vi "updatePerturbation.vi"(6 "delta(T)/baseline(F)":bool, 7 "motor":i32, 8 "timeInterval":dbl, 9 "PertSign":i32, 10 "newValue":dbl, 11 "perturbationIn":T1) -> (3 "perturbationOut":T1)   [LabVIEW 2019]
uses:
  TypeDefs/PerturbationControl.ctl
panel:
  # "This VI is used to update the Perturbation Array inserting newValue in the appropriate cell (based on motor axis, pert sign, pert time, delta or baseline)."
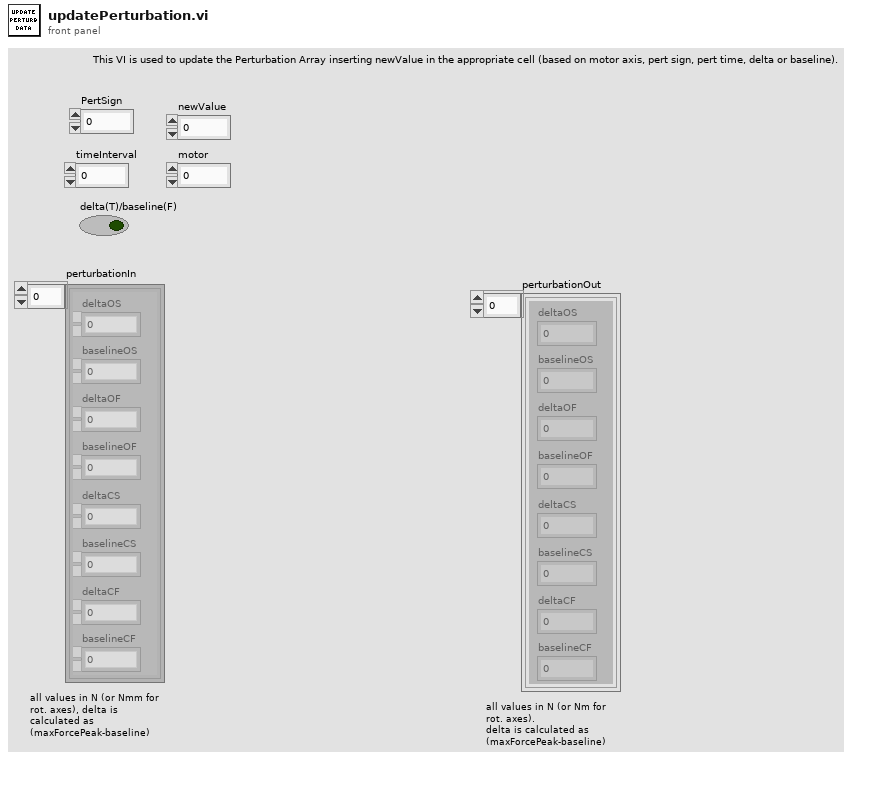
[diagram p1: front panel]
types:
  T1 = typedef "PerturbationControl.ctl" = cluster{"deltaOS":dbl, "baselineOS":dbl, "deltaOF":dbl, "baselineOF":dbl, "deltaCS":dbl, "baselineCS":dbl, "deltaCF":dbl, "baselineCF":dbl}[]
  T2 = cluster{"deltaOS":dbl, "baselineOS":dbl, "deltaOF":dbl, "baselineOF":dbl, "deltaCS":dbl, "baselineCS":dbl, "deltaCF":dbl, "baselineCF":dbl}
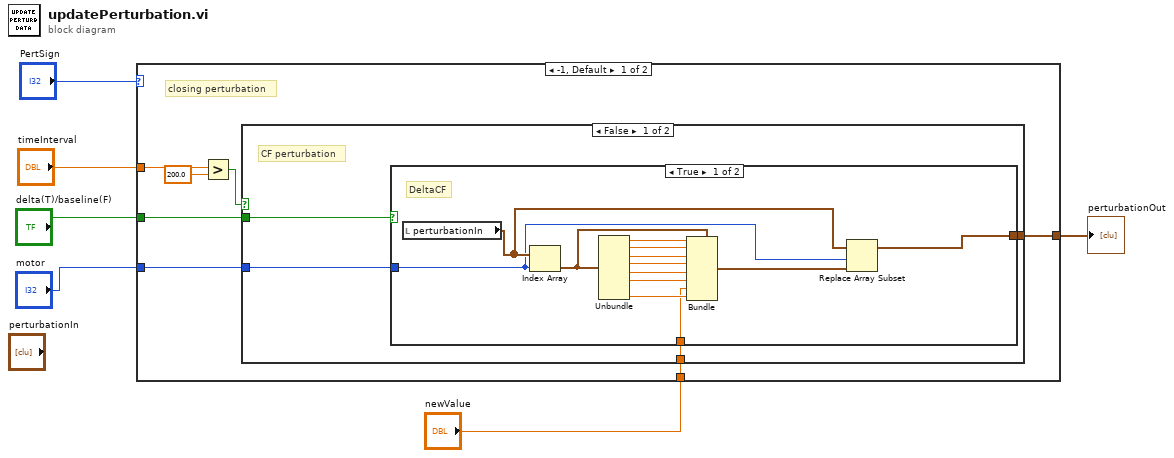
[diagram p0: block diagram]
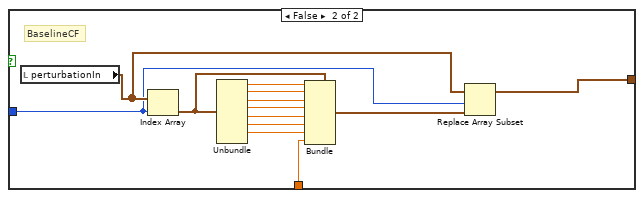
[diagram p2: hidden frame]
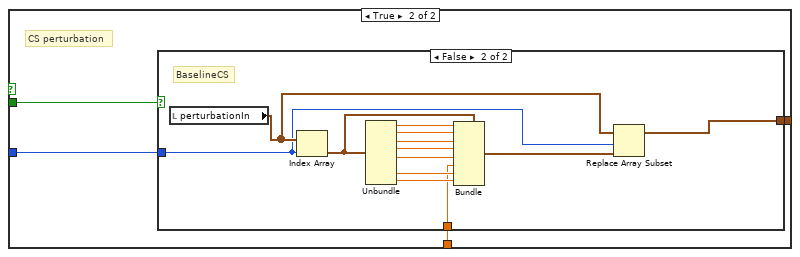
[diagram p3: hidden frame]
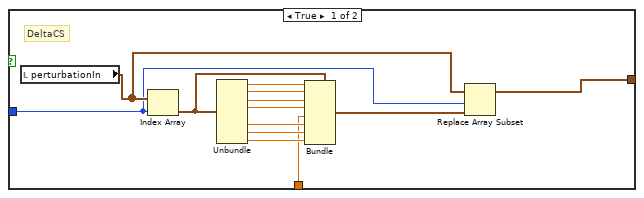
[diagram p4: hidden frame]
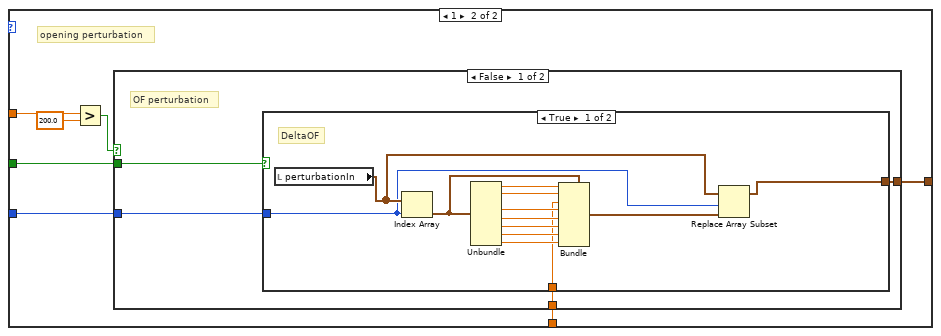
[diagram p5: hidden frame]
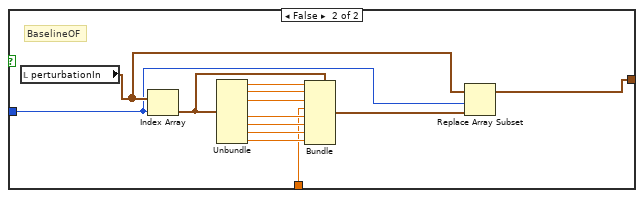
[diagram p6: hidden frame]
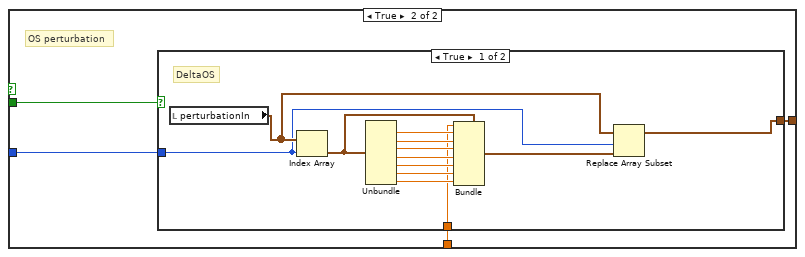
[diagram p7: hidden frame]
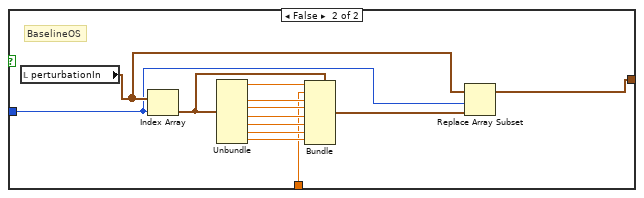
[diagram p8: hidden frame]
diagram:
  n1 = case shown="-1, Default" "PertSign" {
    tunnel: "timeInterval" -> [w13 w80]
    tunnel: "delta(T)/baseline(F)" -> [w10 w77]
    tunnel: "motor" -> [w9 w76]
    tunnel: "newValue" -> [w8 w75]
    tunnel: [w7 w74] -> w1
    frame -1, Default {
      # "closing perturbation"
      n2 = Greater?(x=w13, y=200.0) -> (0:w11:bool)
      n3 = case shown="False" w11 {
        tunnel: w10 -> [w17 w47]
        tunnel: w9 -> [w16 w46]
        tunnel: w8 -> [w15 w45]
        tunnel: [w14 w44] -> w7
        frame False {
          # "CF perturbation"
          n4 = case shown="True" w17 {
            tunnel: w16 -> [w20 w35]
            tunnel: w15 -> [w22 w32]
            tunnel: [w18 w31] -> w14
            frame True {
              # "DeltaCF"
              n5 = local read "perturbationIn"() -> (w21:T1)
              n6 = Index Array(array=w21, index=w20) -> (element=w30:T2)
              n7 = Unbundle(w30) -> ("deltaOS"=w29:dbl, "baselineOS"=w28:dbl, "deltaOF"=w27:dbl, "baselineOF"=w26:dbl, "deltaCS"=w25:dbl, "baselineCS"=w24:dbl, "baselineCF"=w23:dbl)  [unwired: 1 out]
              n8 = Bundle(cluster=w30, "deltaOS"=w29, "baselineOS"=w28, "deltaOF"=w27, "baselineOF"=w26, "deltaCS"=w25, "baselineCS"=w24, "deltaCF"=w22, "baselineCF"=w23) -> (w19:T2)
              n9 = Replace Array Subset(array=w21, new element=w19, index=w20) -> (w18:T1)
            }
            frame False {
              # "BaselineCF"
              n10 = local read "perturbationIn"() -> (w36:T1)
              n11 = Index Array(array=w36, index=w35) -> (element=w43:T2)
              n12 = Unbundle(w43) -> ("deltaOS"=w42:dbl, "baselineOS"=w41:dbl, "deltaOF"=w40:dbl, "baselineOF"=w39:dbl, "deltaCS"=w38:dbl, "baselineCS"=w37:dbl, "deltaCF"=w33:dbl)  [unwired: 1 out]
              n13 = Bundle(cluster=w43, "deltaOS"=w42, "baselineOS"=w41, "deltaOF"=w40, "baselineOF"=w39, "deltaCS"=w38, "baselineCS"=w37, "deltaCF"=w33, "baselineCF"=w32) -> (w34:T2)
              n14 = Replace Array Subset(array=w36, new element=w34, index=w35) -> (w31:T1)
            }
          }
        }
        frame True {
          # "CS perturbation"
          n15 = case shown="False" w47 {
            tunnel: w46 -> [w52 w66]
            tunnel: w45 -> [w49 w62]
            tunnel: [w48 w61] -> w44
            frame True {
              # "DeltaCS"
              n16 = local read "perturbationIn"() -> (w53:T1)
              n17 = Index Array(array=w53, index=w52) -> (element=w60:T2)
              n18 = Unbundle(w60) -> ("deltaOS"=w59:dbl, "baselineOS"=w58:dbl, "deltaOF"=w57:dbl, "baselineOF"=w56:dbl, "baselineCS"=w55:dbl, "deltaCF"=w50:dbl, "baselineCF"=w54:dbl)  [unwired: 1 out]
              n19 = Bundle(cluster=w60, "deltaOS"=w59, "baselineOS"=w58, "deltaOF"=w57, "baselineOF"=w56, "deltaCS"=w49, "baselineCS"=w55, "deltaCF"=w50, "baselineCF"=w54) -> (w51:T2)
              n20 = Replace Array Subset(array=w53, new element=w51, index=w52) -> (w48:T1)
            }
            frame False {
              # "BaselineCS"
              n21 = local read "perturbationIn"() -> (w67:T1)
              n22 = Index Array(array=w67, index=w66) -> (element=w73:T2)
              n23 = Unbundle(w73) -> ("deltaOS"=w72:dbl, "baselineOS"=w71:dbl, "deltaOF"=w70:dbl, "baselineOF"=w69:dbl, "deltaCS"=w68:dbl, "deltaCF"=w64:dbl, "baselineCF"=w63:dbl)  [unwired: 1 out]
              n24 = Bundle(cluster=w73, "deltaOS"=w72, "baselineOS"=w71, "deltaOF"=w70, "baselineOF"=w69, "deltaCS"=w68, "baselineCS"=w62, "deltaCF"=w64, "baselineCF"=w63) -> (w65:T2)
              n25 = Replace Array Subset(array=w67, new element=w65, index=w66) -> (w61:T1)
            }
          }
        }
      }
    }
    frame 1 {
      # "opening perturbation"
      n26 = Greater?(x=w80, y=200.0) -> (0:w78:bool)
      n27 = case shown="False" w78 {
        tunnel: w77 -> [w84 w114]
        tunnel: w76 -> [w83 w113]
        tunnel: w75 -> [w82 w112]
        tunnel: [w81 w111] -> w74
        frame False {
          # "OF perturbation"
          n28 = case shown="True" w84 {
            tunnel: w83 -> [w89 w103]
            tunnel: w82 -> [w86 w99]
            tunnel: [w85 w98] -> w81
            frame True {
              # "DeltaOF"
              n29 = local read "perturbationIn"() -> (w90:T1)
              n30 = Index Array(array=w90, index=w89) -> (element=w97:T2)
              n31 = Unbundle(w97) -> ("deltaOS"=w96:dbl, "baselineOS"=w95:dbl, "baselineOF"=w94:dbl, "deltaCS"=w93:dbl, "baselineCS"=w92:dbl, "deltaCF"=w87:dbl, "baselineCF"=w91:dbl)  [unwired: 1 out]
              n32 = Bundle(cluster=w97, "deltaOS"=w96, "baselineOS"=w95, "deltaOF"=w86, "baselineOF"=w94, "deltaCS"=w93, "baselineCS"=w92, "deltaCF"=w87, "baselineCF"=w91) -> (w88:T2)
              n33 = Replace Array Subset(array=w90, new element=w88, index=w89) -> (w85:T1)
            }
            frame False {
              # "BaselineOF"
              n34 = local read "perturbationIn"() -> (w104:T1)
              n35 = Index Array(array=w104, index=w103) -> (element=w110:T2)
              n36 = Unbundle(w110) -> ("deltaOS"=w109:dbl, "baselineOS"=w108:dbl, "deltaOF"=w107:dbl, "deltaCS"=w106:dbl, "baselineCS"=w105:dbl, "deltaCF"=w101:dbl, "baselineCF"=w100:dbl)  [unwired: 1 out]
              n37 = Bundle(cluster=w110, "deltaOS"=w109, "baselineOS"=w108, "deltaOF"=w107, "baselineOF"=w99, "deltaCS"=w106, "baselineCS"=w105, "deltaCF"=w101, "baselineCF"=w100) -> (w102:T2)
              n38 = Replace Array Subset(array=w104, new element=w102, index=w103) -> (w98:T1)
            }
          }
        }
        frame True {
          # "OS perturbation"
          n39 = case shown="True" w114 {
            tunnel: w113 -> [w120 w134]
            tunnel: w112 -> [w116 w129]
            tunnel: [w115 w128] -> w111
            frame True {
              # "DeltaOS"
              n40 = local read "perturbationIn"() -> (w121:T1)
              n41 = Index Array(array=w121, index=w120) -> (element=w127:T2)
              n42 = Unbundle(w127) -> ("baselineOS"=w126:dbl, "deltaOF"=w125:dbl, "baselineOF"=w124:dbl, "deltaCS"=w117:dbl, "baselineCS"=w123:dbl, "deltaCF"=w118:dbl, "baselineCF"=w122:dbl)  [unwired: 1 out]
              n43 = Bundle(cluster=w127, "deltaOS"=w116, "baselineOS"=w126, "deltaOF"=w125, "baselineOF"=w124, "deltaCS"=w117, "baselineCS"=w123, "deltaCF"=w118, "baselineCF"=w122) -> (w119:T2)
              n44 = Replace Array Subset(array=w121, new element=w119, index=w120) -> (w115:T1)
            }
            frame False {
              # "BaselineOS"
              n45 = local read "perturbationIn"() -> (w135:T1)
              n46 = Index Array(array=w135, index=w134) -> (element=w140:T2)
              n47 = Unbundle(w140) -> ("deltaOS"=w139:dbl, "deltaOF"=w138:dbl, "baselineOF"=w137:dbl, "deltaCS"=w136:dbl, "baselineCS"=w130:dbl, "deltaCF"=w132:dbl, "baselineCF"=w131:dbl)  [unwired: 1 out]
              n48 = Bundle(cluster=w140, "deltaOS"=w139, "baselineOS"=w129, "deltaOF"=w138, "baselineOF"=w137, "deltaCS"=w136, "baselineCS"=w130, "deltaCF"=w132, "baselineCF"=w131) -> (w133:T2)
              n49 = Replace Array Subset(array=w135, new element=w133, index=w134) -> (w128:T1)
            }
          }
        }
      }
    }
  }
  "perturbationOut" <- w1
